vi "REMOND Studio_pH Water Q.vi"() -> ()   [LabVIEW 2021]
uses:
  FSM_States.ctl
  Global_Message.ctl
  <vilib>/Utility/error.llb/DialogType.ctl
  <vilib>/Modbus/master/Modbus Master.lvclass
  Global_flags.vi
  <vilib>/Modbus/master/Create Master Instance (Serial).vi
panel:
  in  "D.S":u16(ring)=1 items=["0.5s", "1s", "1.5s", "2.0s", "2.5s", "3.0s", "3.5s", "4.0s", "4.5s", "5.0s"]
  in  "Measure Mode":u16(ring) items=["[pH]", "[ORP]"]
  in  "Confirm Slope":bool
  in  "Confirm Zero":bool
  out "ADC":u16
  in  "Start Calib":bool
  out "Mensaje de Alarma (Warning):":string
  in  "Exit":bool
  in  "Restore Default":bool
  out "Measurement [pH  ; ORP]:":sgl format="%#.2f pH"
  out "Current Out Val:":sgl format="%#.3f"
  out "Temperature [°C]:":sgl format="%#.1f °C"
  in  "SetBaudRate":bool
  in  "BaudRate (9600)":u16(ring)=2 items=["2400", "4800", "9600", "19200", "38400"]
  in  "BaudRate (9600)":u32=9600
  in  "Addr Set":u16=1 max=255 step=1
  in  "SetAddress":bool
  in  "Address":u8=1
  in  "Standrd Slop Sol.":u16(ring)=1 items=["pH=1.68", "pH=4.01", "pH=9.18", "pH=10.1", "pH=12.45"]
  in  "Set Slope":bool
  in  "Standard Zero Sol.":u16(ring) items=["pH=7.00", "pH=6.86"]
  in  "Set Zero":bool
  in  "Adquire / Stop":bool
  in  "Open/Close COM":bool
  in  "COM":refnum<visa-resource-name>
  out "date /time string":string
  out "Consumer Shutdown?":bool
  # "Calibracion"
  # "Tiempo actual:"
  # "Muestra ADC"
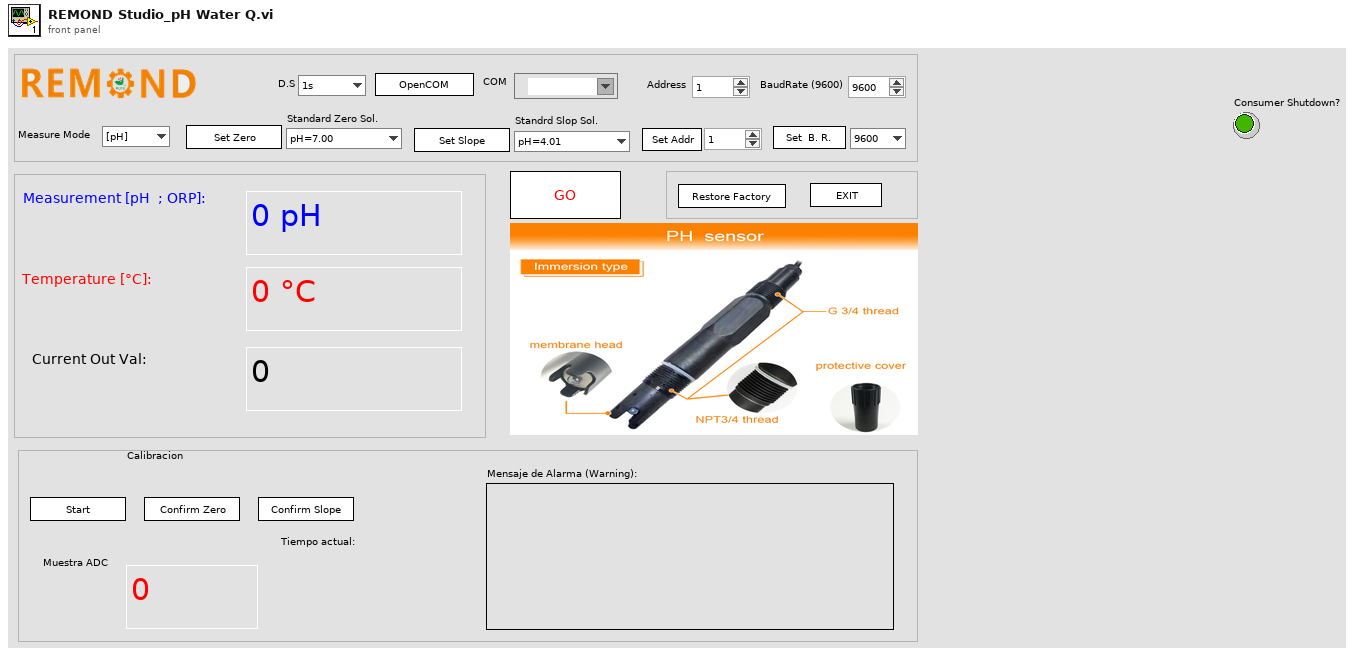
[diagram p1: front panel]
types:
  T1 = typedef "Global_Message.ctl" = cluster{"Consumer State":T2, "User Msg":string, "error in (no error)":errorcluster, "User Msg 2":string}
  T2 = typedef "FSM_States.ctl" = enum16{"Set Measure Mode", "Initialize", "Open COM Port", "Adquire Data", "Set Address", "Set BaudRate", "Restore Factory", "Pre-Set Zero", "Pre-Set K=1", "Pre-Set Slope", "Confirm Zero", "Confirm Slope", "Confirm EC", "Close COM Port", "Exit App", "Stop Data", "Calibrate sensor"}
  T3 = typedef "DialogType.ctl" = u16
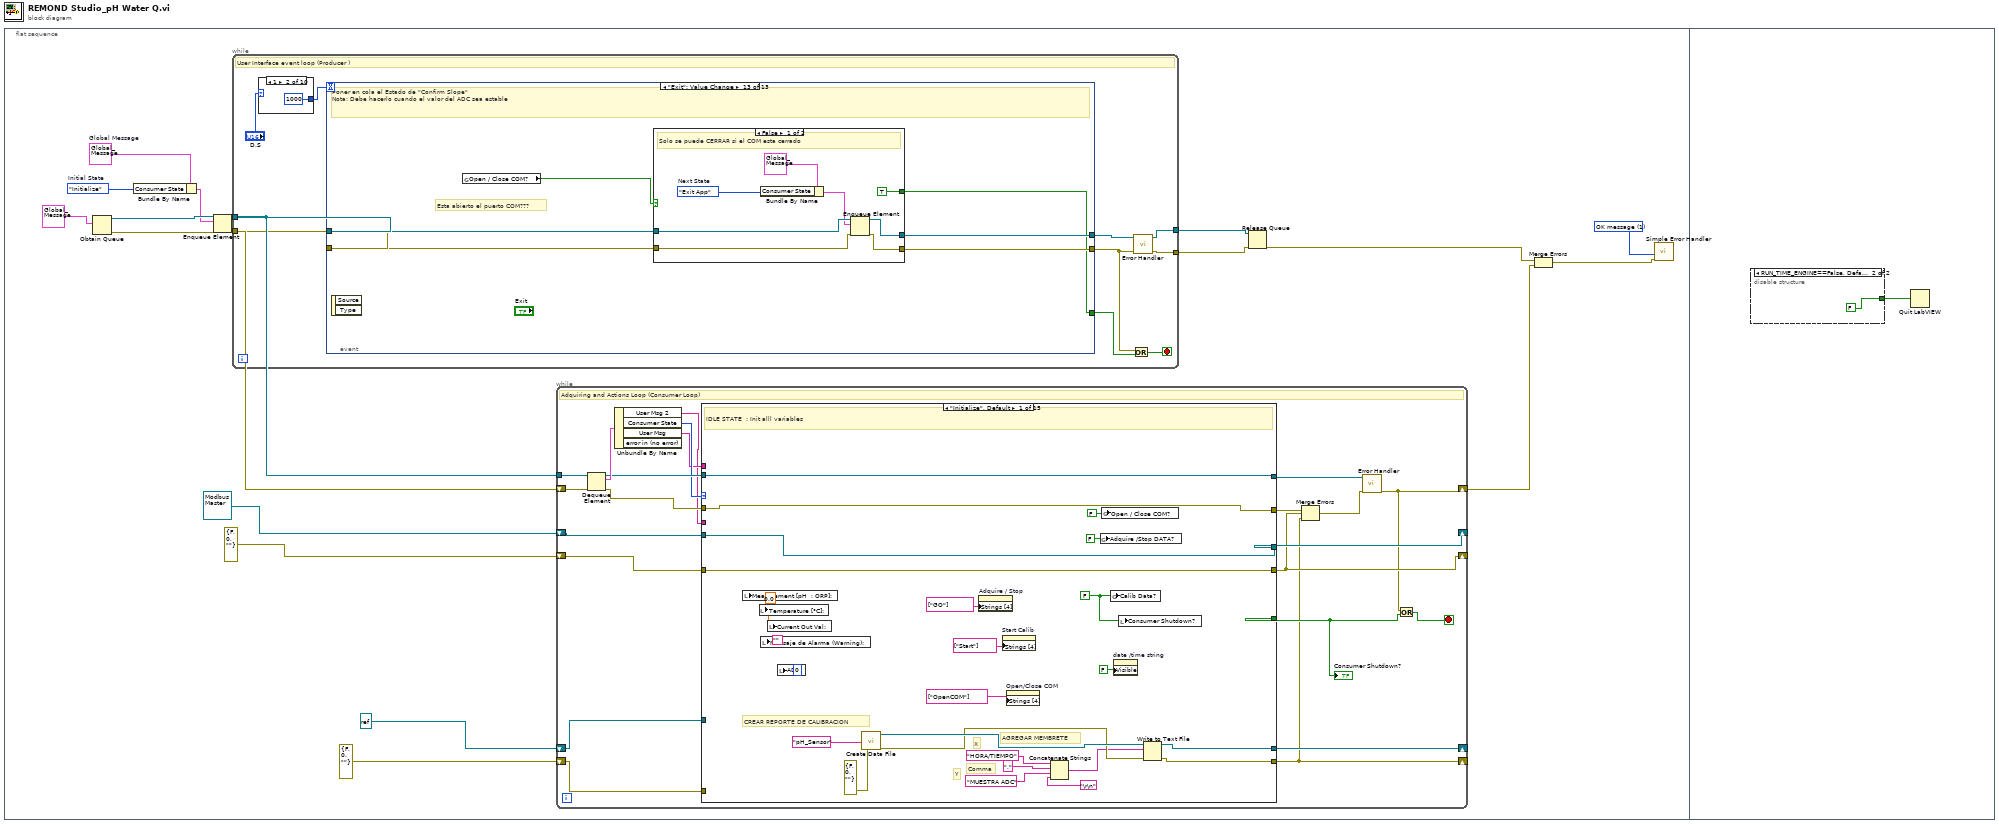
[diagram p0: block diagram]
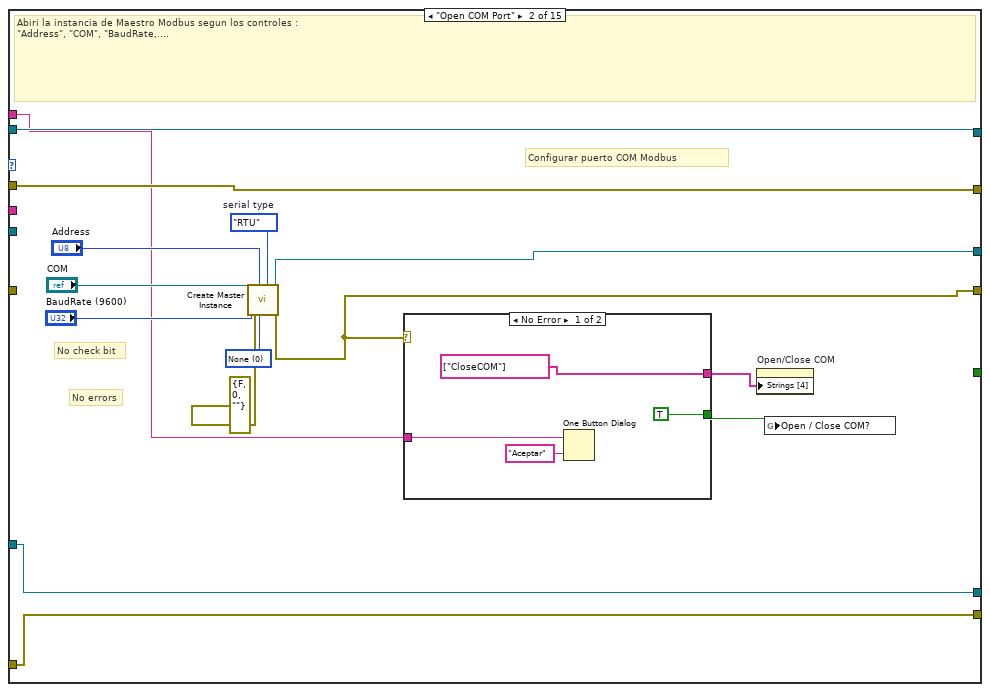
[diagram p2: hidden frame]
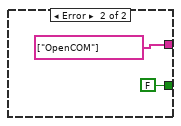
[diagram p3: hidden frame]
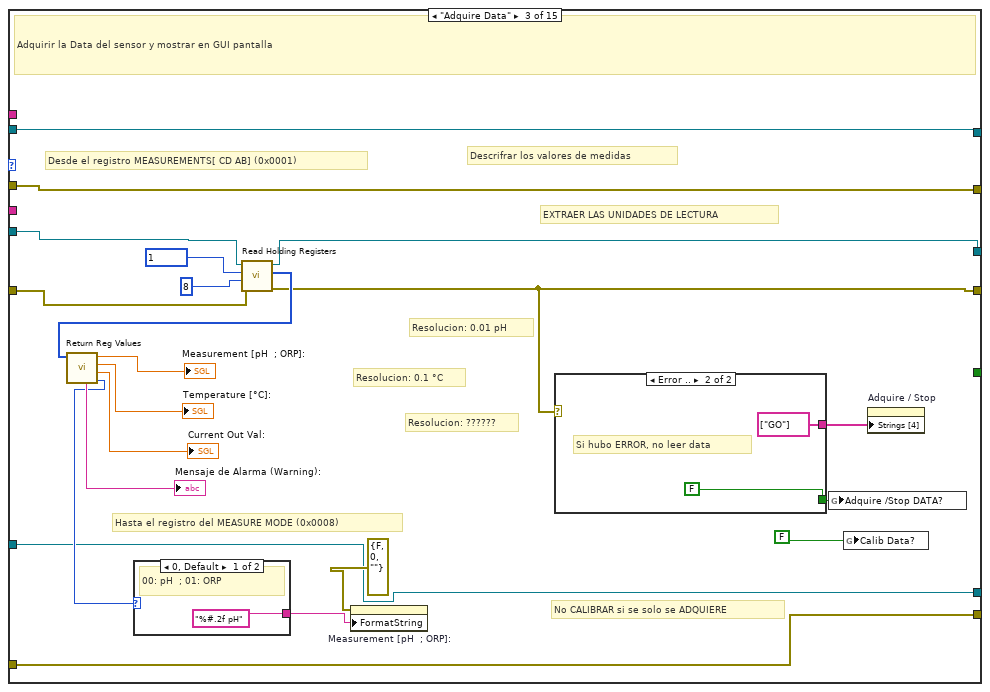
[diagram p4: hidden frame]
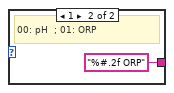
[diagram p5: hidden frame]
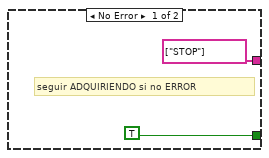
[diagram p6: hidden frame]
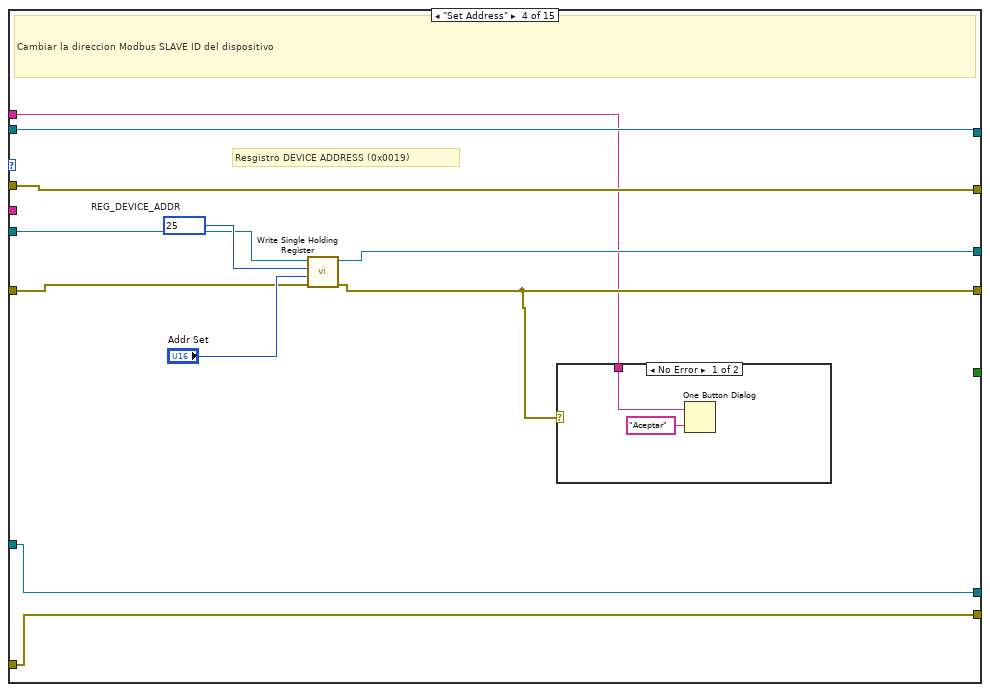
[diagram p7: hidden frame]
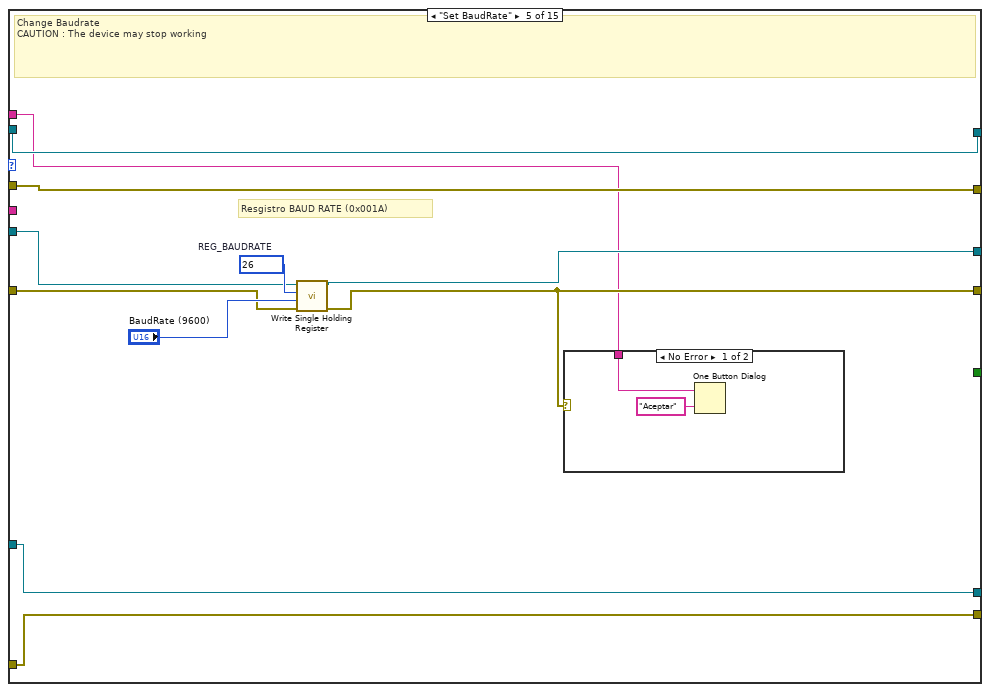
[diagram p9: hidden frame]
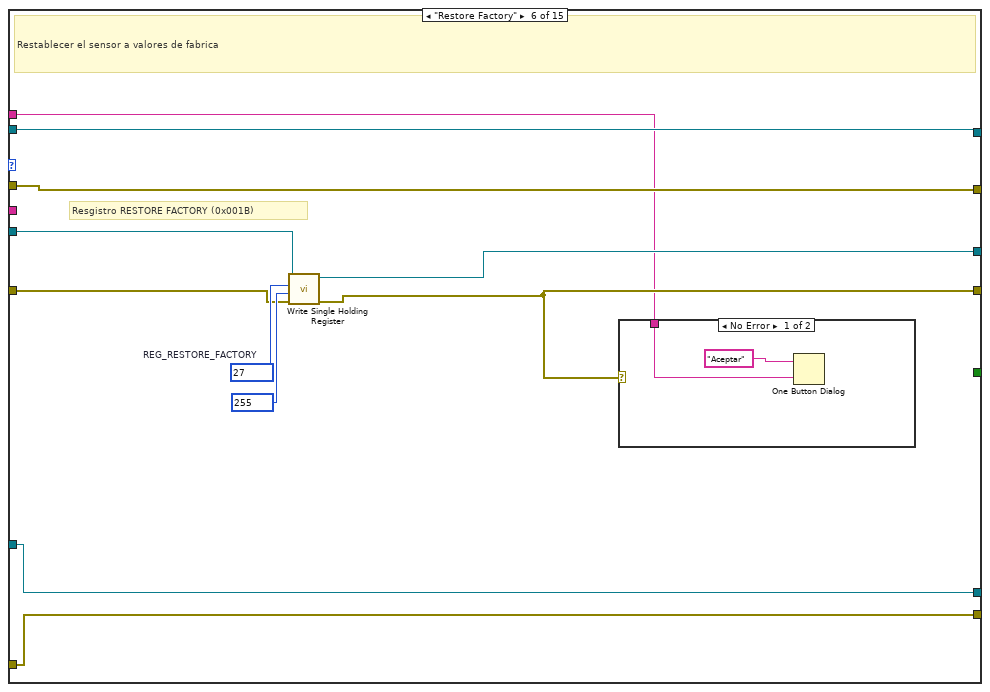
[diagram p11: hidden frame]
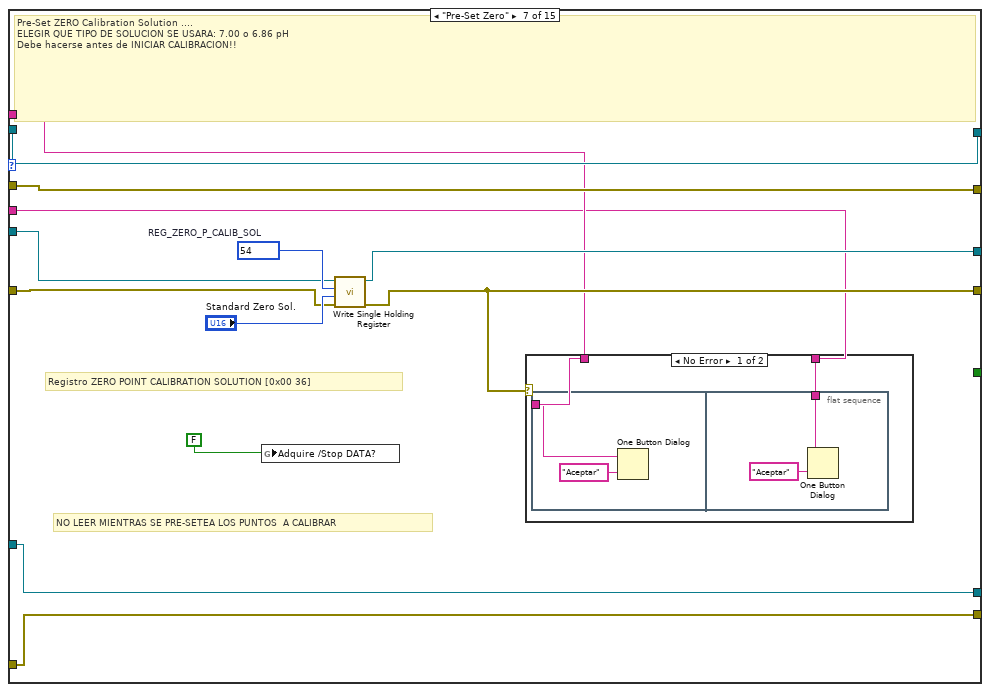
[diagram p13: hidden frame]
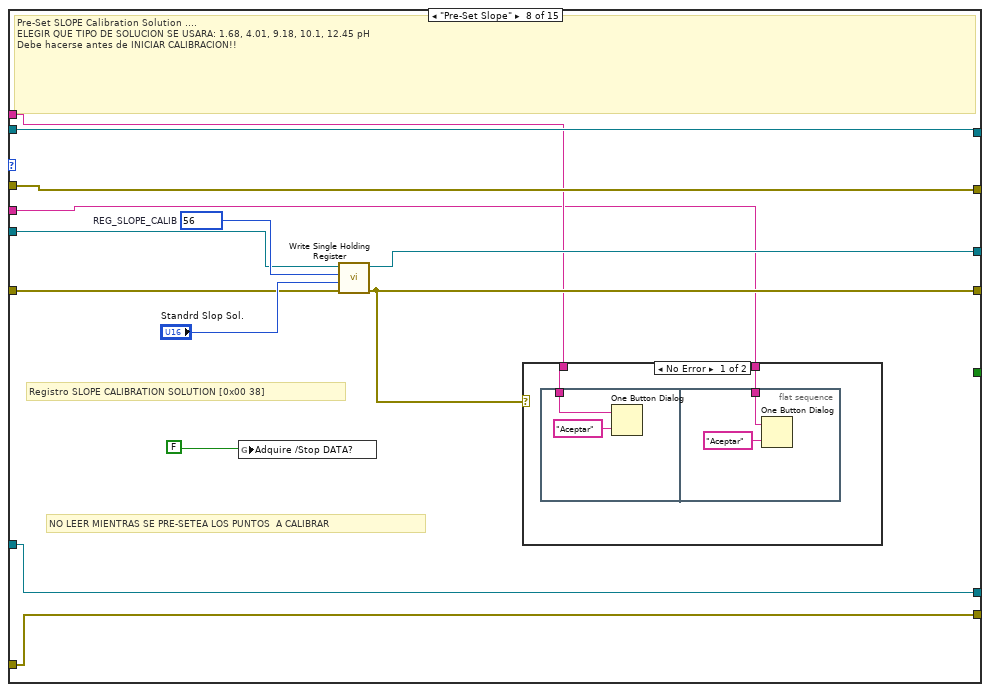
[diagram p15: hidden frame]
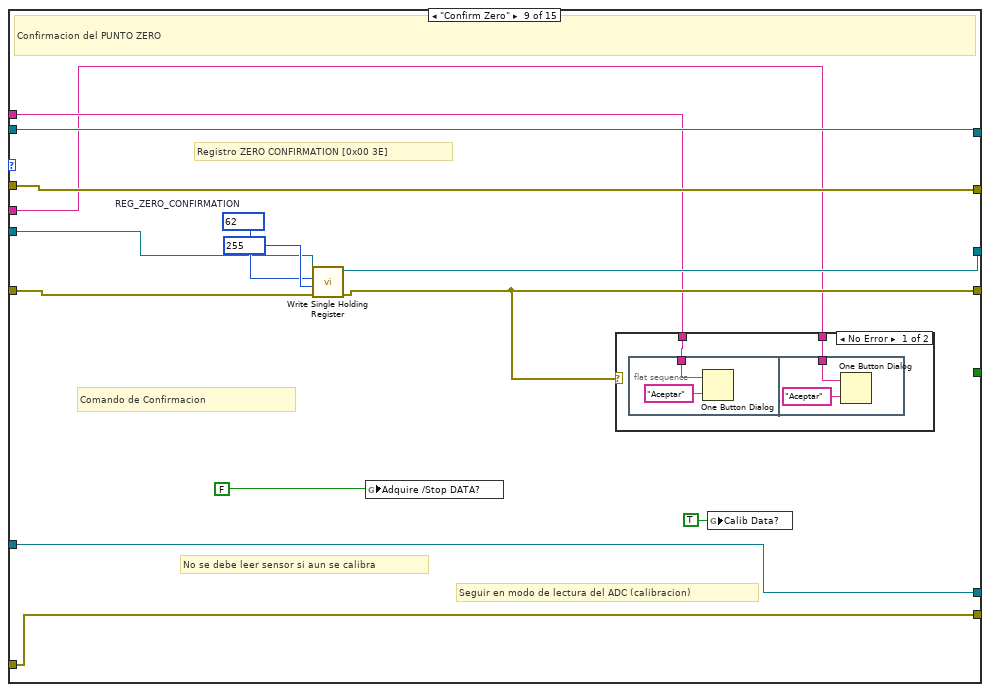
[diagram p17: hidden frame]
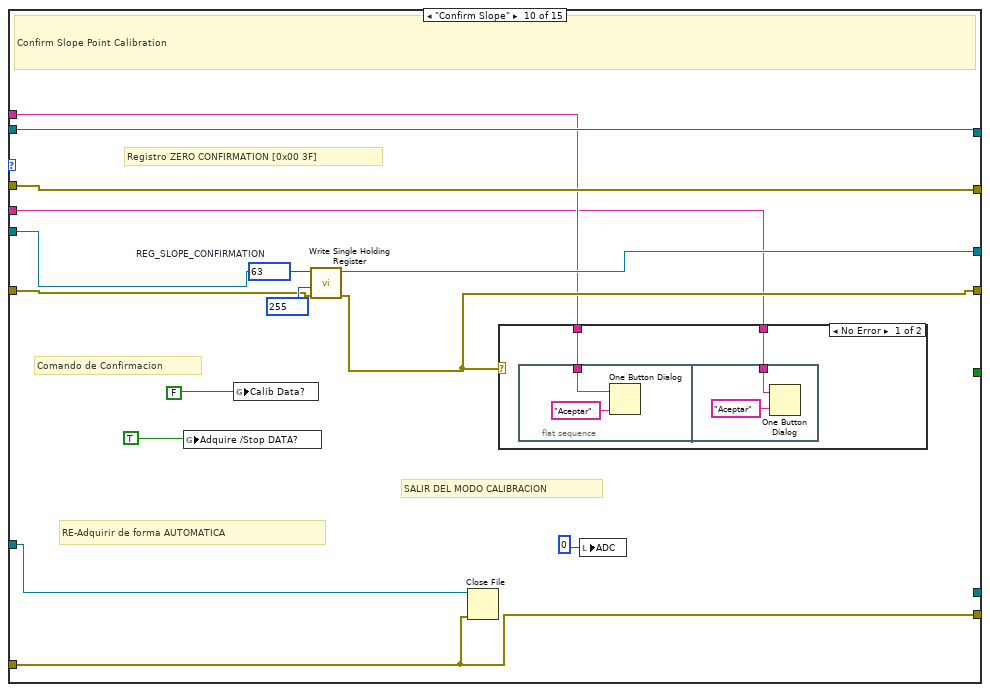
[diagram p19: hidden frame]
diagram:
  n1 = flat-sequence {
    frame #0 {
      w9 = T3 1 items=["no dialog", "OK message", "continue or stop message", "OK message + warnings", "continue/stop + warnings"] ("type of dialog (OK msg:1)")
      w17 = T1 {"Consumer State"=enum."Open COM Port", "User Msg"="", "error in (no error)"={"status"=FALSE, "code"=0, "source"=""}, "User Msg 2"=""}  # Global Message
      w16 = FSM_States."Initialize"  # Initial State
      n2 = Obtain Queue(element data type=T1 {"Consumer State"=enum."Open COM Port", "User Msg"="", "error in (no error)"={"status"=FALSE, "code"=0, "source"=""}, "User Msg 2"=""} ("Global Message")) -> (queue out=w15:refnum<queue>, error out=w14:errorcluster)  [unwired: 4 in, 1 out]
      n3 = Bundle By Name(cluster=w17, "Consumer State"=w16) -> (w13:T1)
      n4 = Enqueue Element(queue=w15, element=w13, error in (no error)=w14) -> (queue out=w11:refnum<queue>, error out=w12:errorcluster)  [unwired: 1 in, 1 out]
      n5 = while {
        tunnel: w11 -> [w321]
        tunnel: w12 -> [w320]
        tunnel: [w318] -> w6
        tunnel: [w317] -> w5
        stop <- w314 stop-if-true
        # "User Interface event loop (Producer )"
        n6 = case shown="1" "D.S" {
          tunnel: [500 1000 1500 2000 2500 3000 3500 4000 4500 5000] -> w312
          frame 0, Default {
          }
          frame 1 {
          }
          frame 2 {
          }
          frame 3 {
          }
          frame 4 {
          }
          frame 5 {
          }
          frame 6 {
          }
          frame 7 {
          }
          frame 8 {
          }
          frame 9 {
          }
        }
        n7 = event shown="[12] \"Exit\": Value Change" {
          selector: _ -> [_ _ _ _ _ _ _ _ _ _ _ _ _]
          dyn-events: _ -> [_ _ _ _ _ _ _ _ _ _ _ _ _]
          timeout: w312 -> [_ _ _ _ _ _ _ _ _ _ _ _ _]
          tunnel: w321 -> [w340 w349 w378 w383 w405 w441 w461 w481 w501 w525 w546 w578 w616]
          tunnel: w320 -> [w339 w348 w377 w382 w403 w440 w460 w480 w500 w524 w545 w577 w615]
          tunnel: [w332 _ _ _ _ _ _ _ _ _ _ _ w611] -> w315
          tunnel: [w338 w347 w374 w381 w404 w439 w459 w479 w499 w523 w544 w579 w614] -> w319
          tunnel: [w337 w346 w373 w380 w402 w438 w458 w478 w498 w522 w543 w576 w613] -> w316
          event Timeout {
            w335 = FSM_States."Stop Data"  # Next State
            w334 = FSM_States."Calibrate sensor"  # Next State
            w343 = FSM_States."Adquire Data"  # Next State
            # "Si ambos flag son FALSE--->>>DETIENE EL MUESTREO"
            # "Si el Flag de CALIB es TRUE-->>>CALIBRAR SENSOR"
            # "Si el Flag de ADQ es TRUE-->>>LEER SENSOR"
            # "Hidden Indicator as Local\nvariable only"
            # "Poner en cola el estado de \"ADQUIRE DATA\" / CALIB DATA de forma automatica cada 1000 mseg(default)"
            n8 = event-data() -> ()  [unwired: 1 in, 1 out]
            n9 = global read "Global_flags.vi" "Adquire /Stop DATA?"() -> (w344:bool)
            n10 = global read "Global_flags.vi" "Calib Data?"() -> (w336:bool)
            n11 = Select(t=w334, s=w336, f=w335) -> (s? t:f=w333:T2)
            n12 = Select(t=w343, s=w344, f=w333) -> (s? t:f=w342:T2)
            n13 = Bundle By Name(cluster=T1 {"Consumer State"=enum."Open COM Port", "User Msg"="", "error in (no error)"={"status"=FALSE, "code"=0, "source"=""}, "User Msg 2"=""} ("Global Message"), "Consumer State"=w342) -> (w341:T1)
            n14 = Enqueue Element(queue=w340, element=w341, error in (no error)=w339) -> (queue out=w338:refnum<queue>, error out=w337:errorcluster)  [unwired: 1 in, 1 out]
            n15 = local read "Consumer Shutdown?"() -> (w332:bool)
          }
          event "Measure Mode": Value Change {
            # "Esta abierto el puerto COM???"
            # "Poner en cola en estado de SET MEASURE MODE (setear en que unidad se toman las muestras)"
            n16 = event-data() -> ()  [unwired: 1 in, 3 out]
            n17 = global read "Global_flags.vi" "Open / Close COM?"() -> (w350:bool)
            n18 = case shown="True" w350 {
              tunnel: w349 -> [w357 w365]
              tunnel: w348 -> [w356 w364]
              tunnel: [w357 w363] -> w347
              tunnel: [w356 w362] -> w346
              frame False {
                # "Solo se puede SET MEASURE si el COM esta abierto"
                n19 = Concatenate Strings("Para cambiar MEASURE MODE::::::" ("message"), "\r\n", "Debe ABRIR Puerto COM !!!" ("string")) -> (w351:string)
                n20 = One Button Dialog(message=w351, button name ("OK")="Aceptar") -> ()  [unwired: 1 out]
              }
              frame True {
                w360 = FSM_States."Set Measure Mode"  # Next State
                # "Solo se puede SET MEASURE si el COM esta abierto"
                n21 = Bundle By Name(cluster=T1 {"Consumer State"=enum."Open COM Port", "User Msg"="", "error in (no error)"={"status"=FALSE, "code"=0, "source"=""}, "User Msg 2"=""} ("Global Message"), "Consumer State"=w360, "User Msg"="OK Measure Mode Changed!!! !!") -> (w359:T1)
                n22 = Enqueue Element(queue=w365, element=w359, error in (no error)=w364) -> (queue out=w363:refnum<queue>, error out=w362:errorcluster)  [unwired: 1 in, 1 out]
              }
            }
          }
          event "Open/Close COM": Value Change {
            w372 = FSM_States."Close COM Port"  # Next State
            w371 = FSM_States."Open COM Port"  # Next State
            # "Poner en cola en estado de apertura de puerto COM Modbus"
            n23 = event-data() -> ()  [unwired: 1 in, 2 out]
            n24 = global read "Global_flags.vi" "Open / Close COM?"() -> (w369:bool)
            n25 = Select(t="Puerto COM cerrado !", s=w369, f="Puerto COM abierto !" ("User Msg")) -> (s? t:f=w366:string)
            n26 = Select(t=w372, s=w369, f=w371) -> (s? t:f=w370:T2)
            n27 = Bundle By Name(cluster=T1 {"Consumer State"=enum."Open COM Port", "User Msg"="", "error in (no error)"={"status"=FALSE, "code"=0, "source"=""}, "User Msg 2"=""} ("Global Message"), "Consumer State"=w370, "User Msg"=w366) -> (w375:T1)
            n28 = Enqueue Element(queue=w378, element=w375, error in (no error)=w377) -> (queue out=w374:refnum<queue>, error out=w373:errorcluster)  [unwired: 1 in, 1 out]
          }
          event "Adquire / Stop": Value Change {
            # "Esta abierto el puerto COM???"
            # "Poner en cola en estado de adquisicion de muestras"
            n29 = event-data() -> ()  [unwired: 1 in, 2 out]
            n30 = global read "Global_flags.vi" "Open / Close COM?"() -> (w379:bool)
            n31 = case shown="True" w379 {
              tunnel: w383 -> [w390 w399]
              tunnel: w382 -> [w389 w398]
              tunnel: [w390 w396] -> w381
              tunnel: [w389 w395] -> w380
              frame False {
                # "Solo se puede ADQUIRIR si el COM esta abierto"
                n32 = Concatenate Strings("Para ADQUIRI muestras::::::" ("message"), "\r\n", "Debe ABRIR Puerto COM !!!" ("string")) -> (w384:string)
                n33 = One Button Dialog(message=w384, button name ("OK")="Aceptar") -> ()  [unwired: 1 out]
              }
              frame True {
                w392 = FSM_States."Adquire Data"  # Next State
                w393 = FSM_States."Stop Data"  # Next State
                # "Si ya se estaba adquiriendo, detener la toma de data"
                # "Solo se puede ADQUIRIR si el COM esta abierto"
                n34 = global read "Global_flags.vi" "Adquire /Stop DATA?"() -> (w391:bool)
                n35 = Select(t=w393, s=w391, f=w392) -> (s? t:f=w394:T2)
                n36 = Bundle By Name(cluster=T1 {"Consumer State"=enum."Open COM Port", "User Msg"="", "error in (no error)"={"status"=FALSE, "code"=0, "source"=""}, "User Msg 2"=""} ("Global Message"), "Consumer State"=w394) -> (w397:T1)
                n37 = Enqueue Element(queue=w399, element=w397, error in (no error)=w398) -> (queue out=w396:refnum<queue>, error out=w395:errorcluster)  [unwired: 1 in, 1 out]
              }
            }
          }
          event "Start Calib": Value Change {
            # "Esta abierto el puerto COM???"
            # "Poner en cola en Estado de \"Start Calibration\""
            n38 = event-data() -> ()  [unwired: 1 in, 2 out]
            n39 = global read "Global_flags.vi" "Open / Close COM?"() -> (w401:bool)
            n40 = case shown="True" w401 {
              tunnel: w405 -> [w412 w416]
              tunnel: [w412 w415] -> w404
              tunnel: w403 -> [w411 w414]
              tunnel: [w411 w413] -> w402
              frame False {
                # "Solo se puede START CALIB si el COM esta abierto"
                n41 = Concatenate Strings("Para EMPEZAR CALIBRACION::::::" ("message"), "\r\n", "Debe ABRIR Puerto COM !!!" ("string")) -> (w410:string)
                n42 = One Button Dialog(message=w410, button name ("OK")="Aceptar") -> ()  [unwired: 1 out]
              }
              frame True {
                # "Solo se puede START CALIB si el COM esta abierto"
                n43 = flat-sequence {
                  tunnel: w414 -> [w425]
                  tunnel: w416 -> [w426]
                  tunnel: [w426] -> w418
                  tunnel: [w425] -> w417
                  tunnel: [w435] -> w415
                  tunnel: [w433] -> w413
                  tunnel: w418 -> [w436]
                  tunnel: w417 -> [w434]
                  frame #0 {
                    w422 = "\r\n"
                    n44 = Concatenate Strings("Modo de calibracion INCIADO! " ("string"), w422, "Nota: Limpiar y sumergir el sensor en  1era Sol. Estand (6.86 o 7.00) [ZERO]" ("string"), w422, "Presione \"Confirm Zero\" cuando la \"Muestra ADC\" sea estable  " ("string")) -> (w420:string)
                    n45 = One Button Dialog(message=w420, button name ("OK")="Aceptar") -> ()  [unwired: 1 out]
                  }
                  frame #1 {
                    w428 = FSM_States."Calibrate sensor"  # Next State
                    w429 = FSM_States."Stop Data"  # Next State
                    # "Si no se esta calibrando  entonces calibrar"
                    n46 = global read "Global_flags.vi" "Calib Data?"() -> (w430:bool)
                    n47 = Select(t=w429, s=w430, f=w428) -> (s? t:f=w427:T2)
                    n48 = Bundle By Name(cluster=T1 {"Consumer State"=enum."Open COM Port", "User Msg"="", "error in (no error)"={"status"=FALSE, "code"=0, "source"=""}, "User Msg 2"=""} ("Global Message"), "Consumer State"=w427) -> (w431:T1)
                    n49 = Enqueue Element At Opposite End(queue=w436, element=w431, error in (no error)=w434) -> (queue out=w435:refnum<queue>, error out=w433:errorcluster)  [unwired: 1 in, 1 out]
                  }
                }
              }
            }
          }
          event "SetAddress": Value Change {
            # "Esta abierto el puerto COM???"
            # "Poner en cola el Estado de Set Address"
            n50 = event-data() -> ()  [unwired: 1 in, 2 out]
            n51 = global read "Global_flags.vi" "Open / Close COM?"() -> (w437:bool)
            n52 = case shown="True" w437 {
              tunnel: w441 -> [w448 w454]
              tunnel: w440 -> [w447 w453]
              tunnel: [w448 w451] -> w439
              tunnel: [w447 w450] -> w438
              frame False {
                # "Solo se puede SET ADDR si el COM esta abierto"
                n53 = Concatenate Strings("Para cambiar SLAVE ID::::::" ("message"), "\r\n", "Debe ABRIR Puerto COM !!!" ("string")) -> (w446:string)
                n54 = One Button Dialog(message=w446, button name ("OK")="Aceptar") -> ()  [unwired: 1 out]
              }
              frame True {
                w455 = FSM_States."Set Address"  # Next State
                # "Solo se puede SET ADDR si el COM esta abierto"
                n55 = Bundle By Name(cluster=T1 {"Consumer State"=enum."Open COM Port", "User Msg"="", "error in (no error)"={"status"=FALSE, "code"=0, "source"=""}, "User Msg 2"=""} ("Global Message"), "Consumer State"=w455, "User Msg"="OK Set Addr !") -> (w452:T1)
                n56 = Enqueue Element(queue=w454, element=w452, error in (no error)=w453) -> (queue out=w451:refnum<queue>, error out=w450:errorcluster)  [unwired: 1 in, 1 out]
              }
            }
          }
          event "SetBaudRate": Value Change {
            # "Esta abierto el puerto COM???"
            # "Poner en cola el Estado de Set Baudrate: Modifica el Baudrate"
            n57 = event-data() -> ()  [unwired: 1 in, 2 out]
            n58 = global read "Global_flags.vi" "Open / Close COM?"() -> (w457:bool)
            n59 = case shown="True" w457 {
              tunnel: w461 -> [w468 w474]
              tunnel: w460 -> [w467 w473]
              tunnel: [w468 w471] -> w459
              tunnel: [w467 w470] -> w458
              frame False {
                # "Solo se puede SetBAUD si el COM esta abierto"
                n60 = Concatenate Strings("Para cambiar BAUDRATE::::::" ("message"), "\r\n", "Debe ABRIR Puerto COM !!!" ("string")) -> (w466:string)
                n61 = One Button Dialog(message=w466, button name ("OK")="Aceptar") -> ()  [unwired: 1 out]
              }
              frame True {
                w475 = FSM_States."Set BaudRate"  # Next State
                # "Solo se puede SetBAUD si el COM esta abierto"
                n62 = Bundle By Name(cluster=T1 {"Consumer State"=enum."Open COM Port", "User Msg"="", "error in (no error)"={"status"=FALSE, "code"=0, "source"=""}, "User Msg 2"=""} ("Global Message"), "Consumer State"=w475, "User Msg"="OK Set Baud !") -> (w472:T1)
                n63 = Enqueue Element(queue=w474, element=w472, error in (no error)=w473) -> (queue out=w471:refnum<queue>, error out=w470:errorcluster)  [unwired: 1 in, 1 out]
              }
            }
          }
          event "Restore Default": Value Change {
            # "Esta abierto el puerto COM???"
            # "Poner en cola el Estado de Restore Default"
            n64 = event-data() -> ()  [unwired: 1 in, 2 out]
            n65 = global read "Global_flags.vi" "Open / Close COM?"() -> (w477:bool)
            n66 = case shown="True" w477 {
              tunnel: w481 -> [w488 w494]
              tunnel: w480 -> [w487 w492]
              tunnel: [w488 w491] -> w479
              tunnel: [w487 w490] -> w478
              frame False {
                # "Solo se puede RESTDEFAULT si el COM esta abierto"
                n67 = Concatenate Strings("Para RESTORE DEFAULT::::::" ("message"), "\r\n", "Debe ABRIR Puerto COM !!!" ("string")) -> (w486:string)
                n68 = One Button Dialog(message=w486, button name ("OK")="Aceptar") -> ()  [unwired: 1 out]
              }
              frame True {
                w495 = FSM_States."Restore Factory"  # Next State
                # "Solo se puede RESTDEFAULT si el COM esta abierto"
                n69 = Bundle By Name(cluster=T1 {"Consumer State"=enum."Open COM Port", "User Msg"="", "error in (no error)"={"status"=FALSE, "code"=0, "source"=""}, "User Msg 2"=""} ("Global Message"), "Consumer State"=w495, "User Msg"="OK Restore Fact !" ("string")) -> (w493:T1)
                n70 = Enqueue Element(queue=w494, element=w493, error in (no error)=w492) -> (queue out=w491:refnum<queue>, error out=w490:errorcluster)  [unwired: 1 in, 1 out]
              }
            }
          }
          event "Set Zero": Value Change {
            # "Esta abierto el puerto COM???"
            # "Poner en cola el Estado de \"Pre-Set-Zero\nNOTA: Debe hacerlo antes de calibrar ADC y tener COM Abierto"
            n71 = event-data() -> ()  [unwired: 1 in, 2 out]
            n72 = global read "Global_flags.vi" "Open / Close COM?"() -> (w497:bool)
            n73 = case shown="True" w497 {
              tunnel: w501 -> [w508 w518]
              tunnel: w500 -> [w507 w517]
              tunnel: [w508 w515] -> w499
              tunnel: [w507 w514] -> w498
              frame False {
                # "Solo se puede SET ZERO si el COM esta abierto"
                n74 = Concatenate Strings("Para SET-ZERO::::::" ("message"), "\r\n", "Debe ABRIR Puerto COM !!!" ("string")) -> (w506:string)
                n75 = One Button Dialog(message=w506, button name ("OK")="Aceptar") -> ()  [unwired: 1 out]
              }
              frame True {
                w519 = FSM_States."Pre-Set Zero"  # Next State
                # "Solo se puede SET ZERO si el COM esta abierto"
                n76 = Concatenate Strings("Ahora haga Clic en \"Set-Slope\"" ("string"), "\r\n", "NOTA: Debe contar con las Sol. Estandar Seleccionado " ("string")) -> (w509:string)
                n77 = Bundle By Name(cluster=T1 {"Consumer State"=enum."Open COM Port", "User Msg"="", "error in (no error)"={"status"=FALSE, "code"=0, "source"=""}, "User Msg 2"=""} ("Global Message"), "Consumer State"=w519, "User Msg"="OK Pre-Set Zero ! ", "User Msg 2"=w509) -> (w516:T1)
                n78 = Enqueue Element(queue=w518, element=w516, error in (no error)=w517) -> (queue out=w515:refnum<queue>, error out=w514:errorcluster)  [unwired: 1 in, 1 out]
              }
            }
          }
          event "Set Slope": Value Change {
            # "Esta abierto el puerto COM???"
            # "Poner en cola el Estado de \"Pre-Set-Slope\nNOTA: Debe hacerlo antes de calibrar ADC y tener COM Abierto"
            n79 = event-data() -> ()  [unwired: 1 in, 2 out]
            n80 = global read "Global_flags.vi" "Open / Close COM?"() -> (w521:bool)
            n81 = case shown="True" w521 {
              tunnel: w525 -> [w532 w539]
              tunnel: w524 -> [w531 w538]
              tunnel: [w532 w536] -> w523
              tunnel: [w531 w535] -> w522
              frame False {
                # "Solo se puede SET SLOPE si el COM esta abierto"
                n82 = Concatenate Strings("Para SET-SLOPE::::::" ("message"), "\r\n", "Debe ABRIR Puerto COM !!!" ("string")) -> (w530:string)
                n83 = One Button Dialog(message=w530, button name ("OK")="Aceptar") -> ()  [unwired: 1 out]
              }
              frame True {
                w540 = FSM_States."Pre-Set Slope"  # Next State
                # "Solo se puede SET SLOPE si el COM esta abierto"
                n84 = Bundle By Name(cluster=T1 {"Consumer State"=enum."Open COM Port", "User Msg"="", "error in (no error)"={"status"=FALSE, "code"=0, "source"=""}, "User Msg 2"=""} ("Global Message"), "Consumer State"=w540, "User Msg"="OK Set Slope !", "User Msg 2"="NOTA: Ahora Presione en \"Start \"Calibracion") -> (w537:T1)
                n85 = Enqueue Element(queue=w539, element=w537, error in (no error)=w538) -> (queue out=w536:refnum<queue>, error out=w535:errorcluster)  [unwired: 1 in, 1 out]
              }
            }
          }
          event "Confirm Zero": Value Change {
            # "Esta abierto el puerto COM???"
            # "Poner en cola el Estado de \"Confirm Zero\"\nNota: Debe hacerlo cuando el valor del ADC sea estable"
            n86 = event-data() -> ()  [unwired: 1 in, 2 out]
            n87 = global read "Global_flags.vi" "Open / Close COM?"() -> (w542:bool)
            n88 = case shown="True" w542 {
              tunnel: w546 -> [w553 w557]
              tunnel: w545 -> [w552 w556]
              tunnel: [w553 w555] -> w544
              tunnel: [w552 w554] -> w543
              frame False {
                # "Solo se puede CONFIRM ZERO si el COM esta abierto"
                n89 = Concatenate Strings("Para CONFIRMAR ZERO::::::" ("message"), "\r\n", "Debe ABRIR Puerto COM Primero !!!" ("string")) -> (w551:string)
                n90 = One Button Dialog(message=w551, button name ("OK")="Aceptar") -> ()  [unwired: 1 out]
              }
              frame True {
                w560 = FSM_States."Stop Data"  # Next State
                w561 = FSM_States."Confirm Zero"  # Next State
                # "Solo se puede CONFIRM ZERO si el COM esta abierto"
                n91 = global read "Global_flags.vi" "Calib Data?"() -> (w559:bool)
                n92 = Select(t=w561, s=w559, f=w560) -> (s? t:f=w558:T2)
                n93 = case shown="True" w559 {
                  tunnel: w558 -> [_ w573]
                  tunnel: w557 -> [w563 w572]
                  tunnel: w556 -> [w562 w571]
                  tunnel: [w563 w570] -> w555
                  tunnel: [w562 w569] -> w554
                  frame False {
                    # "Solo se puede hacer Confirmacion ZERO si se ha estado calibrando !!"
                    n94 = One Button Dialog(message="Para Confirmar ZERO, debe \"START\" Calibracion primero !", button name ("OK")="Aceptar") -> ()  [unwired: 1 out]
                  }
                  frame True {
                    # "Solo se puede hacer Confirmacion ZERO si se ha estado calibrando !!"
                    n95 = Bundle By Name(cluster=T1 {"Consumer State"=enum."Open COM Port", "User Msg"="", "error in (no error)"={"status"=FALSE, "code"=0, "source"=""}, "User Msg 2"=""} ("Global Message"), "Consumer State"=w573, "User Msg"="OK ZERO Confirmado!", "User Msg 2"="Nota: Ahora Limpie y sumerga el sensor en la 2da Sol Estandar(4.01, 10.1, 9.18,etc)  [SLOPE]" ("string")) -> (w568:T1)
                    n96 = Enqueue Element At Opposite End(queue=w572, element=w568, error in (no error)=w571) -> (queue out=w570:refnum<queue>, error out=w569:errorcluster)  [unwired: 1 in, 1 out]
                  }
                }
              }
            }
          }
          event "Confirm Slope": Value Change {
            # "Esta abierto el puerto COM???"
            # "Poner en cola el Estado de \"Confirm Slope\"\nNota: Debe hacerlo cuando el valor del ADC sea estable"
            n97 = event-data() -> ()  [unwired: 1 in, 2 out]
            n98 = global read "Global_flags.vi" "Open / Close COM?"() -> (w575:bool)
            n99 = case shown="True" w575 {
              tunnel: [w586 w591] -> w579
              tunnel: w578 -> [w586 w590]
              tunnel: w577 -> [w585 w589]
              tunnel: [w585 w587] -> w576
              frame False {
                # "Solo se puede CONFIRM ZERO si el COM esta abierto"
                n100 = Concatenate Strings("Para CONFIRMAR SLOPE::::::" ("message"), "\r\n", "Debe ABRIR Puerto COM Primero !!!" ("string")) -> (w584:string)
                n101 = One Button Dialog(message=w584, button name ("OK")="Aceptar") -> ()  [unwired: 1 out]
              }
              frame True {
                w593 = FSM_States."Stop Data"  # Next State
                w594 = FSM_States."Confirm Slope"  # Next State
                # "Estamos CALIBRANDO??"
                # "Solo se puede CONFIRM ZERO si el COM esta abierto"
                n102 = global read "Global_flags.vi" "Calib Data?"() -> (w592:bool)
                n103 = Select(t=w594, s=w592, f=w593) -> (s? t:f=w588:T2)
                n104 = case shown="True" w592 {
                  tunnel: [w596 w610] -> w591
                  tunnel: w590 -> [w596 w609]
                  tunnel: w589 -> [w595 w608]
                  tunnel: w588 -> [_ w605]
                  tunnel: [w595 w604] -> w587
                  frame False {
                    # "Solo se puede hacer Confirmacion SLOPE si se ha estado calibrando !!"
                    n105 = One Button Dialog(message="Para Confirmar Slope, debe \"START\" Calibracion primero !", button name ("OK")="Aceptar") -> ()  [unwired: 1 out]
                  }
                  frame True {
                    # "Solo se puede hacer Confirmacion si se ha estado calibrando !!"
                    n106 = Concatenate Strings("FIN de la calibracion:::::::::::" ("string"), "\r\n", "MODO de Lectura RE-establecido !!!!" ("string")) -> (w599:string)
                    n107 = Bundle By Name(cluster=T1 {"Consumer State"=enum."Open COM Port", "User Msg"="", "error in (no error)"={"status"=FALSE, "code"=0, "source"=""}, "User Msg 2"=""} ("Global Message"), "Consumer State"=w605, "User Msg"="OK SLOPE confirmado !", "User Msg 2"=w599) -> (w606:T1)
                    n108 = Enqueue Element At Opposite End(queue=w609, element=w606, error in (no error)=w608) -> (queue out=w610:refnum<queue>, error out=w604:errorcluster)  [unwired: 1 in, 1 out]
                  }
                }
              }
            }
          }
          event "Exit": Value Change {
            # "Esta abierto el puerto COM???"
            # "Poner en cola el Estado de \"Confirm Slope\"\nNota: Debe hacerlo cuando el valor del ADC sea estable"
            n109 = event-data() -> ()  [unwired: 1 in, 2 out]
            n110 = global read "Global_flags.vi" "Open / Close COM?"() -> (w612:bool)
            n111 = case shown="False" w612 {
              tunnel: w616 -> [w622 w627]
              tunnel: w615 -> [w621 w626]
              tunnel: [w619 w627] -> w614
              tunnel: [w618 w626] -> w613
              tunnel: [TRUE FALSE] -> w611
              frame False {
                w623 = FSM_States."Exit App"  # Next State
                # "Solo se puede CERRAR si el COM esta cerrado"
                n112 = Bundle By Name(cluster=T1 {"Consumer State"=enum."Open COM Port", "User Msg"="", "error in (no error)"={"status"=FALSE, "code"=0, "source"=""}, "User Msg 2"=""} ("Global Message"), "Consumer State"=w623) -> (w620:T1)
                n113 = Enqueue Element(queue=w622, element=w620, error in (no error)=w621) -> (queue out=w619:refnum<queue>, error out=w618:errorcluster)  [unwired: 1 in, 1 out]
              }
              frame True {
                # "Solo se puede CERRAR si el COM esta cerrado"
                n114 = Concatenate Strings("No puede CERRAR::::::" ("message"), "\r\n", "Esta Abierto el  Puerto COM !!!" ("string")) -> (w632:string)
                n115 = One Button Dialog(message=w632, button name ("OK")="Aceptar") -> ()  [unwired: 1 out]
              }
            }
          }
        }
        n116 = Or(x=w316, y=w315) -> (x .or. y?=w314:bool)
        n117 = call "Error Handler.vi"("error in (no error)"=w316, "Queue in"=w319) -> ("error out"=w317:errorcluster, "Queue out"=w318:refnum<queue>)  [unwired: 8 in]
      }
      n118 = while {
        tunnel: w11 -> [w40]
        shift-right: [w37] -> _
        shift-left: refnum<class "Modbus Master.lvclass"> refnum ("Modbus master out") -> [w36]
        shift-right: [w29] -> _
        shift-left: errorcluster {"status"=FALSE, "code"=0, "source"=""} ("error constant") -> [w35]
        shift-right: [w28] -> w10
        shift-left: w12 -> [w39]
        shift-right: [w22] -> _
        shift-left: refnum<file> refnum ("refnum out") -> [w21]
        shift-right: [w19] -> _
        shift-left: errorcluster {"status"=FALSE, "code"=0, "source"=""} ("error out") -> [w20]
        stop <- w26 stop-if-true
        # "Adquiring and Actions Loop (Consumer Loop)"
        n119 = Dequeue Element(queue=w40, error in (no error)=w39) -> (queue out=w32:refnum<queue>, element=w38:T1, error out=w34:errorcluster)  [unwired: 1 in, 1 out]
        n120 = Unbundle By Name(w38) -> ("User Msg 2"=w23:string, "Consumer State"=w25:T2, "User Msg"=w24:string)  [unwired: 1 out]
        n121 = case shown="\"Initialize\", Default" w25 {
          tunnel: [w65 w74 w102 w121 w134 w147 w161 w181 w200 w221 _ _ w265 w287 w304] -> w37
          tunnel: [w64 w69 w96 w117 w130 w143 w158 w177 w197 w216 w237 _ w264 w280 w302] -> w29
          tunnel: w36 -> [w65 _ w103 w122 w135 w148 w163 w182 w202 w223 w241 _ w265 w288 w306]
          tunnel: w35 -> [w64 _ w101 w120 w133 w146 w162 w180 w201 w222 w240 w250 w264 w286 w305]
          tunnel: [_ _ _ _ _ _ _ _ _ _ _ TRUE _ _ _] -> w27
          tunnel: w34 -> [w54 w70 w98 w118 w131 w144 w159 w178 w198 w217 w238 w251 w259 w282 w308]
          tunnel: [w55 w71 w99 w119 w132 w145 w160 w179 w199 w218 w239 w248 w260 w283 w309] -> w33
          tunnel: w32 -> [w55 w71 w99 w119 w132 w145 w160 w179 w199 w218 w239 w248 w260 w283 w309]
          tunnel: [w54 w70 w98 w118 w131 w144 w159 w178 w198 w217 w238 w247 w259 w282 w308] -> w31
          tunnel: w24 -> [_ w68 _ w116 w129 w142 w157 w176 w196 w215 w234 _ _ _ w301]
          tunnel: w23 -> [_ _ _ _ _ _ w155 w174 w193 w213 _ _ _ _ _]
          tunnel: [w43 w67 w89 w115 w128 w141 w154 w173 w192 _ w233 _ w254 w277 w300] -> w22
          tunnel: [w42 w66 w88 w114 w127 w140 w153 w172 w191 w211 w232 w244 w253 w276 w299] -> w19
          tunnel: w21 -> [_ w67 w89 w115 w128 w141 w154 w173 w192 w212 w233 w246 w254 w267 w300]
          tunnel: w20 -> [_ w66 w88 w114 w127 w140 w153 w172 w191 w211 w232 w245 w253 w266 w299]
          frame "Initialize", Default {
            w56 = FALSE ("Adquire /Stop DATA?")
            w63 = sgl 0.0 ("pH:")
            # "Comma"
            # "Y"
            # "AGREGAR MEMBRETE"
            # "X"
            # "CREAR REPORTE DE CALIBRACION"
            # "IDLE STATE  : Init alll variables"
            n122 = local write "Measurement [pH  ; ORP]:"(w63) -> ()
            n123 = local write "Temperature [°C]:"(w63) -> ()
            n124 = local write "Mensaje de Alarma (Warning):"("") -> ()
            n125 = local write "Current Out Val:"(w63) -> ()
            n126 = local write "ADC"(u16 0 ("ADC")) -> ()
            n127 = call "Create Data File.vi"("error in"=errorcluster {"status"=FALSE, "code"=0, "source"=""}, "UUT"="pH_Sensor") -> ("error out"=w45:errorcluster, "refnum out"=w46:refnum<file>)  [unwired: 8 in]
            n128 = property on="Adquire / Stop" class="Bool"("Strings [4]"=string[] ["GO"]) -> ()  [unwired: 2 in, 2 out]
            n129 = property on="Start Calib" class="Bool"("Strings [4]"=string[] ["Start"]) -> ()  [unwired: 2 in, 2 out]
            n130 = property on="Open/Close COM" class="Bool"("Strings [4]"=string[] ["OpenCOM"]) -> ()  [unwired: 2 in, 2 out]
            n131 = Concatenate Strings("HORA/TIEMPO" ("string"), "," ("string"), "MUESTRA ADC" ("string"), "\r\n") -> (w44:string)
            n132 = global write "Global_flags.vi" "Adquire /Stop DATA?"(FALSE ("Adquire /Stop DATA?")) -> ()
            n133 = global write "Global_flags.vi" "Open / Close COM?"(FALSE ("Open / Close COM?")) -> ()
            n134 = global write "Global_flags.vi" "Calib Data?"(w56) -> ()
            n135 = property on="date /time string" class="Str"("Visible"=FALSE) -> ()  [unwired: 2 in, 2 out]
            n136 = local write "Consumer Shutdown?"(w56) -> ()
            n137 = Write to Text File(file (use dialog)=w46, text=w44, error in=w45) -> (refnum out=w43:refnum<file>, error out=w42:errorcluster)  [unwired: 1 in, 1 out]
          }
          frame "Open COM Port" {
            w76 = u16 0 items=["None", "Odd", "Even"] ("parity (Even)")
            w77 = enum16{"RTU", "ASCII"}."RTU"  # serial type
            # "Configurar puerto COM Modbus"
            # "No errors"
            # "No check bit"
            # "Abiri la instancia de Maestro Modbus segun los controles : \n\"Address\", \"COM\", \"BaudRate,...."
            n138 = call-poly <vilib>:"Create Master Instance.vi"("serial type"=w77, "parity (Even)"=w76, "unit ID"="Address", "error in (no error)"=errorcluster {"status"=FALSE, "code"=0, "source"=""}, "baud rate (9600)"="BaudRate (9600)", "VISA resource name"="COM") -> ("error out"=w69:errorcluster, "serial master instance"=w74:refnum<class "Modbus Master.lvclass">)  [unwired: 4 in]
            n139 = case shown="No Error" w69 {
              tunnel: [string[] ["CloseCOM"] ("Strings [4]") string[] ["OpenCOM"] ("Strings [4]")] -> w73
              tunnel: [TRUE FALSE] -> w72
              tunnel: w68 -> [w82 _]
              frame No Error {
                n140 = One Button Dialog(message=w82, button name ("OK")="Aceptar") -> ()  [unwired: 1 out]
              }
              frame Error {
              }
            }
            n141 = property on="Open/Close COM" class="Bool"("Strings [4]"=w73) -> ()  [unwired: 2 in, 2 out]
            n142 = global write "Global_flags.vi" "Open / Close COM?"(w72) -> ()
          }
          frame "Adquire Data" {
            # "EXTRAER LAS UNIDADES DE LECTURA"
            # "Resolucion: ??????"
            # "Resolucion: 0.1 °C"
            # "Resolucion: 0.01 pH"
            # "No CALIBRAR si se solo se ADQUIERE"
            # "Descrifrar los valores de medidas"
            # "Hasta el registro del MEASURE MODE (0x0008)"
            # "Desde el registro MEASUREMENTS[ CD AB] (0x0001)"
            # "Adquirir la Data del sensor y mostrar en GUI pantalla"
            n143 = call-dynamic "Read Holding Registers.vi"("error in (no error)"=w101, "number of holding registers"=u16 8, "starting address"=u16 1, "Modbus master in"=w103) -> ("error out"=w96:errorcluster, "register values"=w106:u16[], "Modbus master out"=w102:refnum<class "Modbus Master.lvclass">)  [unwired: 5 in]
            n144 = call "Return Reg Values.vi"("Register Values"=w106) -> ("Measure Mode"=w92:u16, "Current Output value"=→"Current Out Val:":sgl, "Temperature Measurement"=→"Temperature [°C]:":sgl, "Measurements"=→"Measurement [pH  ; ORP]:":sgl, "Warning"=→"Mensaje de Alarma (Warning):":string)  [unwired: 6 in]
            n145 = case shown="0, Default" w92 {
              tunnel: ["%#.2f pH" "%#.2f ORP"] -> w91
              frame 0, Default {
                # "00: pH  ; 01: ORP"
              }
              frame 1 {
                # "00: pH  ; 01: ORP"
              }
            }
            n146 = property on="Measurement [pH  ; ORP]:" class="DigNum (strict)"(error in=errorcluster {"status"=FALSE, "code"=0, "source"=""} ("error in (no error)"), "FormatString"=w91) -> ()  [unwired: 1 in, 2 out]
            n147 = case shown="Error .." w96 {
              tunnel: [TRUE FALSE] -> w100
              tunnel: [string[] ["STOP"] ("Strings [4]") string[] ["GO"] ("Strings [4]")] -> w87
              frame No Error {
                # "seguir ADQUIRIENDO si no ERROR"
              }
              frame Error {
                # "Si hubo ERROR, no leer data"
              }
            }
            n148 = global write "Global_flags.vi" "Adquire /Stop DATA?"(w100) -> ()
            n149 = global write "Global_flags.vi" "Calib Data?"(FALSE ("Calib Data?")) -> ()
            n150 = property on="Adquire / Stop" class="Bool"("Strings [4]"=w87) -> ()  [unwired: 2 in, 2 out]
          }
          frame "Set Address" {
            w123 = u16 25  # REG_DEVICE_ADDR
            # "Resgistro DEVICE ADDRESS (0x0019)"
            # "Cambiar la direccion Modbus SLAVE ID del dispositivo"
            n151 = call-dynamic "Write Single Holding Register.vi"("error in (no error)"=w120, "holding register value"="Addr Set", "address"=w123, "Modbus master in"=w122) -> ("error out"=w117:errorcluster, "Modbus master out"=w121:refnum<class "Modbus Master.lvclass">)  [unwired: 6 in]
            n152 = case shown="No Error" w117 {
              tunnel: w116 -> [w126 _]
              frame No Error {
                n153 = One Button Dialog(message=w126, button name ("OK")="Aceptar") -> ()  [unwired: 1 out]
              }
              frame Error {
              }
            }
          }
          frame "Set BaudRate" {
            w136 = u16 26  # REG_BAUDRATE
            # "Resgistro BAUD RATE (0x001A)"
            # "Change Baudrate  \nCAUTION : The device may stop working"
            n154 = call-dynamic "Write Single Holding Register.vi"("error in (no error)"=w133, "holding register value"="BaudRate (9600)", "address"=w136, "Modbus master in"=w135) -> ("error out"=w130:errorcluster, "Modbus master out"=w134:refnum<class "Modbus Master.lvclass">)  [unwired: 6 in]
            n155 = case shown="No Error" w130 {
              tunnel: w129 -> [w139 _]
              frame No Error {
                n156 = One Button Dialog(message=w139, button name ("OK")="Aceptar") -> ()  [unwired: 1 out]
              }
              frame Error {
              }
            }
          }
          frame "Restore Factory" {
            w149 = u16 27  # REG_RESTORE_FACTORY
            # "Resgistro RESTORE FACTORY (0x001B)"
            # "Restablecer el sensor a valores de fabrica"
            n157 = call-dynamic "Write Single Holding Register.vi"("error in (no error)"=w146, "holding register value"=u16 255, "address"=w149, "Modbus master in"=w148) -> ("error out"=w143:errorcluster, "Modbus master out"=w147:refnum<class "Modbus Master.lvclass">)  [unwired: 6 in]
            n158 = case shown="No Error" w143 {
              tunnel: w142 -> [w151 _]
              frame No Error {
                n159 = One Button Dialog(message="Aceptar", button name ("OK")=w151) -> ()  [unwired: 1 out]
              }
              frame Error {
              }
            }
          }
          frame "Pre-Set Zero" {
            w164 = u16 54  # REG_ZERO_P_CALIB_SOL
            # "NO LEER MIENTRAS SE PRE-SETEA LOS PUNTOS  A CALIBRAR"
            # "Registro ZERO POINT CALIBRATION SOLUTION [0x00 36]"
            # "Pre-Set ZERO Calibration Solution ....\nELEGIR QUE TIPO DE SOLUCION SE USARA: 7.00 o 6.86 pH\nDebe hacerse antes de INICIAR CALIBRACION!!"
            n160 = global write "Global_flags.vi" "Adquire /Stop DATA?"(FALSE) -> ()
            n161 = call-dynamic "Write Single Holding Register.vi"("error in (no error)"=w162, "holding register value"="Standard Zero Sol.", "address"=w164, "Modbus master in"=w163) -> ("error out"=w158:errorcluster, "Modbus master out"=w161:refnum<class "Modbus Master.lvclass">)  [unwired: 6 in]
            n162 = case shown="No Error" w158 {
              tunnel: w157 -> [w167 _]
              tunnel: w155 -> [w166 _]
              frame No Error {
                n163 = flat-sequence {
                  tunnel: w167 -> [w169]
                  tunnel: w166 -> [w171]
                  frame #0 {
                    n164 = One Button Dialog(message=w169, button name ("OK")="Aceptar") -> ()  [unwired: 1 out]
                  }
                  frame #1 {
                    n165 = One Button Dialog(message=w171, button name ("OK")="Aceptar") -> ()  [unwired: 1 out]
                  }
                }
              }
              frame Error {
              }
            }
          }
          frame "Pre-Set Slope" {
            w183 = u16 56  # REG_SLOPE_CALIB
            # "NO LEER MIENTRAS SE PRE-SETEA LOS PUNTOS  A CALIBRAR"
            # "Registro SLOPE CALIBRATION SOLUTION [0x00 38]"
            # "Pre-Set SLOPE Calibration Solution ....\nELEGIR QUE TIPO DE SOLUCION SE USARA: 1.68, 4.01, 9.18, 10.1, 12.45 pH\nDebe hacerse antes de INICIAR CALIBRACION!!"
            n166 = global write "Global_flags.vi" "Adquire /Stop DATA?"(FALSE) -> ()
            n167 = call-dynamic "Write Single Holding Register.vi"("error in (no error)"=w180, "holding register value"="Standrd Slop Sol.", "address"=w183, "Modbus master in"=w182) -> ("error out"=w177:errorcluster, "Modbus master out"=w181:refnum<class "Modbus Master.lvclass">)  [unwired: 6 in]
            n168 = case shown="No Error" w177 {
              tunnel: w176 -> [w186 _]
              tunnel: w174 -> [w185 _]
              frame No Error {
                n169 = flat-sequence {
                  tunnel: w186 -> [w188]
                  tunnel: w185 -> [w190]
                  frame #0 {
                    n170 = One Button Dialog(message=w188, button name ("OK")="Aceptar") -> ()  [unwired: 1 out]
                  }
                  frame #1 {
                    n171 = One Button Dialog(message=w190, button name ("OK")="Aceptar") -> ()  [unwired: 1 out]
                  }
                }
              }
              frame Error {
              }
            }
          }
          frame "Confirm Zero" {
            w203 = u16 62  # REG_ZERO_CONFIRMATION
            # "Seguir en modo de lectura del ADC (calibracion)"
            # "No se debe leer sensor si aun se calibra"
            # "Comando de Confirmacion"
            # "Registro ZERO CONFIRMATION [0x00 3E]"
            # "Confirmacion del PUNTO ZERO"
            n172 = call-dynamic "Write Single Holding Register.vi"("error in (no error)"=w201, "holding register value"=u16 255 ("address"), "address"=w203, "Modbus master in"=w202) -> ("error out"=w197:errorcluster, "Modbus master out"=w200:refnum<class "Modbus Master.lvclass">)  [unwired: 6 in]
            n173 = global write "Global_flags.vi" "Adquire /Stop DATA?"(FALSE) -> ()
            n174 = case shown="No Error" w197 {
              tunnel: w196 -> [w206 _]
              tunnel: w193 -> [w205 _]
              frame No Error {
                n175 = flat-sequence {
                  tunnel: w206 -> [w208]
                  tunnel: w205 -> [w209]
                  frame #0 {
                    n176 = One Button Dialog(message=w208, button name ("OK")="Aceptar") -> ()  [unwired: 1 out]
                  }
                  frame #1 {
                    n177 = One Button Dialog(message=w209, button name ("OK")="Aceptar") -> ()  [unwired: 1 out]
                  }
                }
              }
              frame Error {
              }
            }
            n178 = global write "Global_flags.vi" "Calib Data?"(TRUE ("Calib Data?")) -> ()
          }
          frame "Confirm Slope" {
            w224 = u16 63  # REG_SLOPE_CONFIRMATION
            # "Registro ZERO CONFIRMATION [0x00 3F]"
            # "SALIR DEL MODO CALIBRACION"
            # "RE-Adquirir de forma AUTOMATICA"
            # "Comando de Confirmacion"
            # "Confirm Slope Point Calibration"
            n179 = global write "Global_flags.vi" "Adquire /Stop DATA?"(TRUE) -> ()
            n180 = global write "Global_flags.vi" "Calib Data?"(FALSE ("Adquire /Stop DATA?")) -> ()
            n181 = call-dynamic "Write Single Holding Register.vi"("error in (no error)"=w222, "holding register value"=u16 255 ("address"), "address"=w224, "Modbus master in"=w223) -> ("error out"=w216:errorcluster, "Modbus master out"=w221:refnum<class "Modbus Master.lvclass">)  [unwired: 6 in]
            n182 = Close File(refnum=w212, error in=w211) -> ()  [unwired: 2 out]
            n183 = case shown="No Error" w216 {
              tunnel: w215 -> [w227 _]
              tunnel: w213 -> [w226 _]
              frame No Error {
                n184 = flat-sequence {
                  tunnel: w227 -> [w228]
                  tunnel: w226 -> [w230]
                  frame #0 {
                    n185 = One Button Dialog(message=w228, button name ("OK")="Aceptar") -> ()  [unwired: 1 out]
                  }
                  frame #1 {
                    n186 = One Button Dialog(message=w230, button name ("OK")="Aceptar") -> ()  [unwired: 1 out]
                  }
                }
              }
              frame Error {
              }
            }
            n187 = local write "ADC"(u16 0 ("ADC")) -> ()
          }
          frame "Close COM Port" {
            # "Closes Serial COM Port"
            n188 = property on="Open/Close COM" class="Bool"("Strings [4]"=string[] ["OpenCOM"]) -> ()  [unwired: 2 in, 2 out]
            n189 = call-dynamic "Close.vi"("error in (no error)"=w240, "Modbus master in"=w241) -> ("error out"=w237:errorcluster)  [unwired: 9 in]
            n190 = global write "Global_flags.vi" "Open / Close COM?"(FALSE ("Open / Close COM?")) -> ()
            n191 = case shown="No Error" w237 {
              tunnel: w234 -> [w243 _]
              frame No Error {
                n192 = One Button Dialog(message=w243, button name ("OK")="Aceptar") -> ()  [unwired: 1 out]
              }
              frame Error {
              }
            }
          }
          frame "Exit App" {
            w249 = T3 3 items=["no dialog", "OK message", "continue or stop message", "OK message + warnings", "continue/stop + warnings"] ("type of dialog (OK msg:1)")
            # "Releases the queue"
            # "Releases queue and EXIT App"
            n193 = Merge Errors(w251, w250) -> (w247:errorcluster)
            n194 = Close File(refnum=w246, error in=w245) -> (error out=w244:errorcluster)  [unwired: 1 out]
            n195 = call <vilib>:"Simple Error Handler.vi"("type of dialog (OK msg:1)"=w249, "error in (no error)"=w247) -> ()  [unwired: 3 in, 5 out]
          }
          frame "Stop Data" {
            w263 = sgl 0.0 ("pH:")
            # "Deja de tomar datos del sensor y pone a 0 los indicadores"
            n196 = local write "Measurement [pH  ; ORP]:"(w263) -> ()
            n197 = local write "Temperature [°C]:"(w263) -> ()
            n198 = local write "Mensaje de Alarma (Warning):"("") -> ()
            n199 = local write "Current Out Val:"(w263) -> ()
            n200 = local write "ADC"(u16 0 ("ADC")) -> ()
            n201 = property on="Adquire / Stop" class="Bool"("Strings [4]"=string[] ["GO"]) -> ()  [unwired: 2 in, 2 out]
            n202 = global write "Global_flags.vi" "Adquire /Stop DATA?"(FALSE ("Adquire /Stop DATA?")) -> ()
            n203 = global write "Global_flags.vi" "Calib Data?"(FALSE) -> ()
            n204 = property on="date /time string" class="Str"("Visible"=FALSE) -> ()  [unwired: 2 in, 2 out]
          }
          frame "Calibrate sensor" {
            w289 = u16 102  # REG_MEASURED_ADC
            # "ESCRIBIR EN REPORTE"
            # "Dato ADC"
            # "comma"
            # "Hora:Minuto:Segundo"
            # "Registro MEASURED ADC [0x00 66]"
            # "No adquirir mientras se calibra"
            # "VALOR ADC"
            # "Leer el valor ADC para poder calibrar"
            n205 = Format Date/Time String(time format string (%c)="%H : %M : %S ") -> (date/time string=→"date /time string":string)  [unwired: 2 in]
            n206 = call-dynamic "Read Holding Registers.vi"("error in (no error)"=w286, "number of holding registers"=u16 1, "starting address"=w289, "Modbus master in"=w288) -> ("error out"=w280:errorcluster, "register values"=w292:u16[], "Modbus master out"=w287:refnum<class "Modbus Master.lvclass">)  [unwired: 5 in]
            n207 = Index Array(array=w292, index=0) -> (element=w270:u16)
            "ADC" <- w270
            n208 = Format Date/Time String(time format string (%c)="%H:%M%S") -> (date/time string=w274:string)  [unwired: 2 in]
            n209 = case shown="No Error" w280 {
              tunnel: [w294 FALSE] -> w281
              tunnel: [w293 FALSE ("Visible")] -> w279
              frame No Error {
                n210 = flat-sequence {
                  tunnel: [TRUE] -> w294
                  tunnel: [TRUE ("Visible")] -> w293
                  frame #0 {
                    # "EMPEZAR A CALIBRAR SENSOR"
                    # "Visible la trama de Tiempo"
                  }
                }
              }
              frame Error {
                # "Si falla , no se calibra"
              }
            }
            n211 = Format Into String(format string="%04d", w270) -> (resulting string=w272:string)  [unwired: 2 in, 1 out]
            n212 = Concatenate Strings(w274, "," ("string"), w272, "\r\n") -> (w268:string)
            n213 = global write "Global_flags.vi" "Adquire /Stop DATA?"(FALSE) -> ()
            n214 = global write "Global_flags.vi" "Calib Data?"(w281) -> ()
            n215 = Write to Text File(file (use dialog)=w267, text=w268, error in=w266) -> (refnum out=w277:refnum<file>, error out=w276:errorcluster)  [unwired: 1 in, 1 out]
            n216 = property on="date /time string" class="Str"("Visible"=w279) -> ()  [unwired: 2 in, 2 out]
          }
          frame "Set Measure Mode" {
            # "Capturar 00 [pH]  o 01[ORP]"
            # "Resgistro MEASUREMENT MODE (0x0008)"
            # "Cambiar el MEASURE MODE  [pH /ORP] del sensor"
            n217 = local read "Measure Mode"() -> (w303:u16)
            n218 = call-dynamic "Write Single Holding Register.vi"("error in (no error)"=w305, "holding register value"=w303, "address"=u16 8, "Modbus master in"=w306) -> ("error out"=w302:errorcluster, "Modbus master out"=w304:refnum<class "Modbus Master.lvclass">)  [unwired: 6 in]
            n219 = case shown="No Error" w302 {
              tunnel: w301 -> [w310 _]
              frame No Error {
                n220 = One Button Dialog(message=w310, button name ("OK")="Aceptar") -> ()  [unwired: 1 out]
              }
              frame Error {
              }
            }
          }
        }
        "Consumer Shutdown?" <- w27
        n221 = Merge Errors(w31, w29, w19) -> (w30:errorcluster)
        n222 = call "Error Handler.vi"("error in (no error)"=w30, "Queue in"=w33) -> ("error out"=w28:errorcluster)  [unwired: 8 in, 1 out]
        n223 = Or(x=w28, y=w27) -> (x .or. y?=w26:bool)
      }
      n224 = Release Queue(queue=w6, error in (no error)=w5) -> (error out=w4:errorcluster)  [unwired: 1 in, 2 out]
      n225 = Merge Errors(w4, w10) -> (w3:errorcluster)
      n226 = call <vilib>:"Simple Error Handler.vi"("type of dialog (OK msg:1)"=w9, "error in (no error)"=w3) -> ()  [unwired: 3 in, 5 out]
    }
    frame #1 {
      n227 = disable-structure shown="RUN_TIME_ENGINE==False, Default" {
        disable-tunnel: [TRUE FALSE] -> w633
        frame condition #0 {
        }
        frame condition #1 (active) {
        }
      }
      n228 = Quit LabVIEW(quit? (T)=w633) -> ()
    }
  }
